vi "Log System Errors to File.vi"(8 "error out":errorcluster, 10 "Comments":string, 11 "Path":path=path "C:/Documents and Settings/Inalfa/Desktop") -> (0 "error out":errorcluster)   [LabVIEW 2015]
uses:
  <vilib>/Utility/file.llb/Read From Spreadsheet File (string).vi
  <vilib>/Utility/file.llb/Write To Spreadsheet File (string).vi
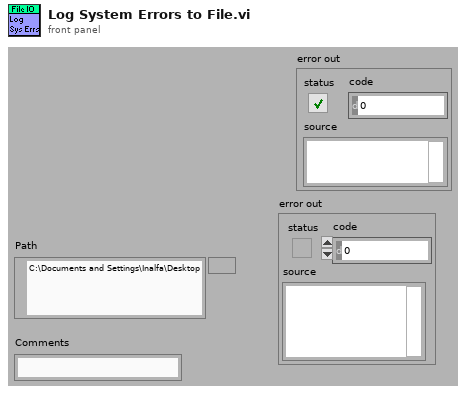
[diagram p1: front panel]
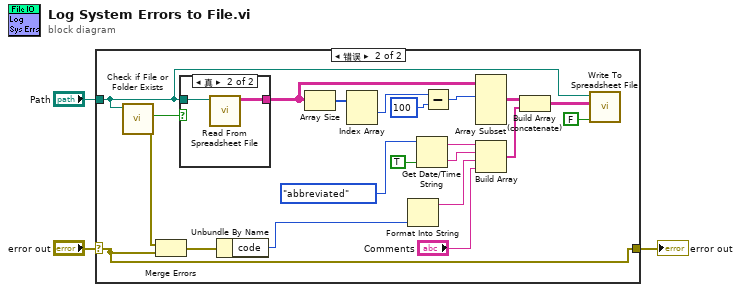
[diagram p0: block diagram]
diagram:
  n1 = case shown="错误" "error out" {
    selector: "error out" -> [w4 w6]
    tunnel: [w4 w6] -> w2
    tunnel: "Path" -> [_ w9]
    frame No Error {
    }
    frame Error {
      n2 = call <vilib>:"Check if File or Folder Exists.vi"("path"=w9) -> ("error out"=w7:errorcluster, "file or folder exists?"=w8:bool)  [unwired: 8 in, 1 out]
      n3 = Merge Errors(w7, w6) -> (w5:errorcluster)
      n4 = case shown="真" w8 {
        tunnel: [_ w27] -> w16
        tunnel: w9 -> [_ w26]
        frame False {
        }
        frame True {
          n5 = call-poly <vilib>:"Read From Spreadsheet File.vi"("file path (dialog if empty)"=w26) -> ("all rows"=w27:string[][])  [unwired: 6 in, 4 out]
        }
      }
      n6 = Unbundle By Name(w5) -> ("code"=w23:i32)
      n7 = Array Size(array=w16) -> (size(s)=w15:i32[])
      n8 = Index Array(array=w15) -> (element #1=w14:i32)  [unwired: 2 in, 1 out]
      n9 = Format Into String(w23) -> (resulting string=w22:string)  [unwired: 3 in, 1 out]
      n10 = Get Date/Time String(date format (0)=enum16{"short", "long", "abbreviated"}."abbreviated", want seconds? (F)=TRUE) -> (date string=w25:string, time string=w24:string)  [unwired: 1 out]
      n11 = Subtract(x=w14, y=100) -> (x-y=w13:i32)
      n12 = Array Subset(array=w16, index (row)=w13) -> (w18:string[][])  [unwired: 3 in]
      n13 = Build Array(w25, w24, w22, "Comments") -> (w19:string[])
      n14 = Build Array (concatenate)(w18, w19) -> (w17:string[][])
      n15 = call-poly <vilib>:"Write To Spreadsheet File.vi"("append to file? (new file:F)"=FALSE, "2D data"=w17, "file path (dialog if empty)"=w9) -> ()  [unwired: 3 in, 3 out]
    }
  }
  "error out" <- w2
